vi "Transfer Sample Get Transfer Controls.vi"(8 "error in (no error)":errorcluster, 11 "cRIO-CO2 in":refnum<class "cRIO-CO2.lvclass">) -> (0 "error out":errorcluster, 1 "Target Container":T1, 2 "Source Container":T1, 3 "cRIO-CO2 out":refnum<class "cRIO-CO2.lvclass">, 4 "Transfer mBar":dbl)   [LabVIEW 2015, in "cRIO-Carbondioxide.lvlib" / "cRIO-CO2.lvlib" / "cRIO-CO2.lvclass"]
uses:
  cRIO-CO2.lvclass
  Controls/Sample Transfer Container Enumerator.ctl
  cRIO-CO2.lvclass/cRIO-CO2.ctl
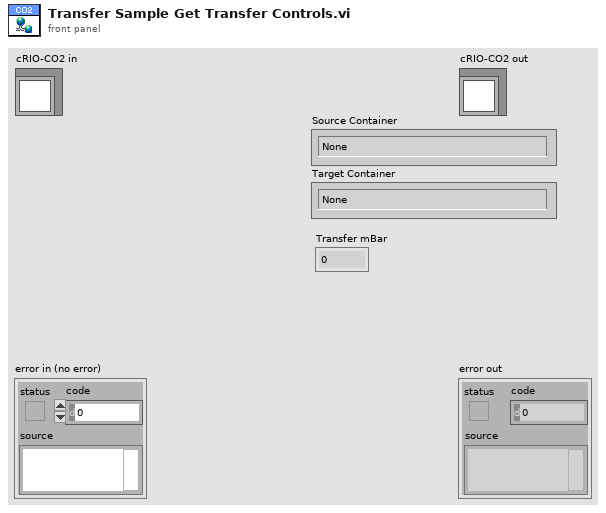
[diagram p1: front panel]
types:
  T1 = typedef "Sample Transfer Container Enumerator.ctl" = enum16{"None", "Sample 1", "Sample 2", "Sample 3", "Sample 4", "Sample 5", "Storage 01", "Storage 02", "Storage 03", "Storage 04", "Storage 05", "Storage 06", "Storage 07", "Storage 08", "Storage 09", "Storage 10", "Storage 11", "Storage 12", "Syringe", "Undefined"}
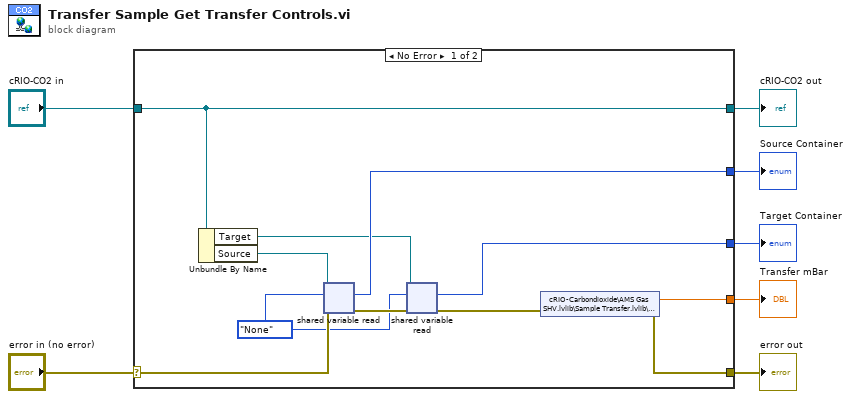
[diagram p0: block diagram]
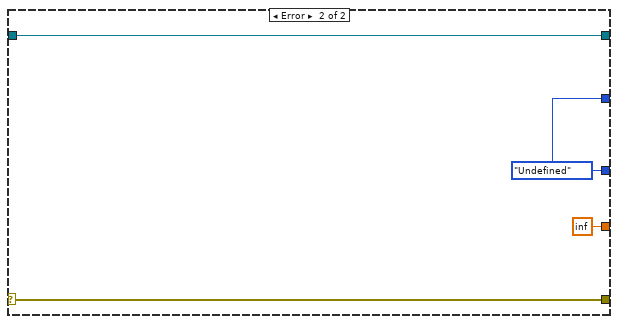
[diagram p2: hidden frame]
diagram:
  n1 = case shown="No Error" "error in (no error)" {
    selector: "error in (no error)" -> [w15 w22]
    tunnel: [w14 w22] -> w6
    tunnel: [w18 w21] -> w4
    tunnel: "cRIO-CO2 in" -> [w18 w21]
    tunnel: [w11 w19] -> w3
    tunnel: [w10 w19] -> w2
    tunnel: [w8 inf ("Double")] -> w1
    frame No Error {
      w13 = Sample_Transfer_Container_Enumerator."None" ("Source Container")
      n2 = Unbundle By Name(w18) -> ("Target"=w9:refnum<k21>, "Source"=w12:refnum<k21>)
      n3 = shared-variable-read(w12, w15, w13) -> (w17:errorcluster, w11:T1)  [unwired: 2 out]
      n4 = shared-variable-read(w9, w17, w13) -> (w16:errorcluster, w10:T1)  [unwired: 2 out]
      n5 = shared-variable "cRIO-Carbondioxide\\AMS Gas SHV.lvlib\\Sample Transfer.lvlib\\Transfer mBar"(error in=w16) -> (w8:dbl, error out=w14:errorcluster)
    }
    frame Error {
      w19 = Sample_Transfer_Container_Enumerator."Undefined" ("Source Container")
    }
  }
  "error out" <- w6
  "cRIO-CO2 out" <- w4
  "Source Container" <- w3
  "Target Container" <- w2
  "Transfer mBar" <- w1
